vi "Refname to String (Other Motors).vi"(1 "Enum":T1) -> (0 "resulting string":string)   [LabVIEW 2016, in "Huskie Swerve.lvlib"]
uses:
  Huskie Swerve.lvlib
  Other Motors.ctl
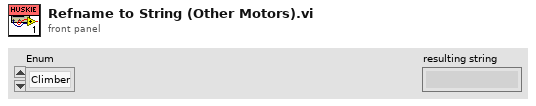
[diagram p1: front panel]
types:
  T1 = typedef "Huskie Swerve.lvlib/Other Motors.ctl" = enum16{"Climber", "Other motor", "Random Motor", "Spinny thingamajig", "Moves some blobs"}
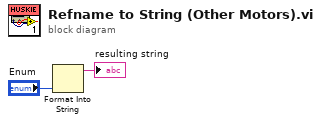
[diagram p0: block diagram]
diagram:
  n1 = Format Into String("Enum") -> (resulting string=→"resulting string":string)  [unwired: 3 in, 1 out]
